vi "RTAF Global References.vi"() -> ()   [LabVIEW 2020]
uses:
  Actors/Logger/API/Logger Actor API.lvclass
  Actors/Alarms Handler/API/Alarms Handler Actor API.lvclass
  Actors/Test/API/Test Actor API.lvclass
  Actors/System Status/API/System Status Actor API.lvclass
panel:
  in  "System Status":refnum<class "System Status Actor API.lvclass">
  in  "Test":refnum<class "Test Actor API.lvclass">
  in  "Alarms Handler":refnum<class "Alarms Handler Actor API.lvclass">
  in  "Logger":refnum<class "Logger Actor API.lvclass">
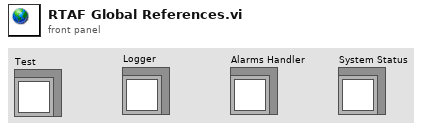
[diagram p1: front panel]
diagram:
